vi "Module Name--constant.vi"() -> (3 "Module Name":string)   [LabVIEW 2020, in "Navigation.lvlib"]
doc: "Return the name of the module that owns this VI. \n____\nHAMPEL SOFTWARE ENGINEERING v2.6.0 (2023-12-19 10:54)"
uses:
  Navigation.lvlib
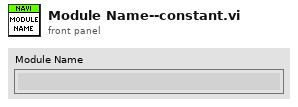
[diagram p1: front panel]
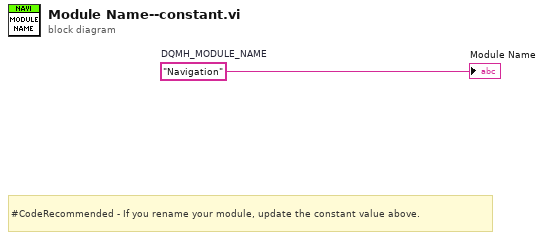
[diagram p0: block diagram]
diagram:
  w1 = "Navigation"  # DQMH_MODULE_NAME
  # "#CodeRecommended - If you rename your module, update the constant value above."
  "Module Name" <- w1
